vi "Calc ScaleFactor.vi"(8 "error in (no error)":errorcluster, 11 "[A/D Input]":dbl[][](array[numeric])) -> (0 "error out":errorcluster, 1 "ScaleFactorB":i32, 2 "ScaleFactorA":i32, 3 "Pass?":bool, 4 "May Pass Retest?":bool, 5 "GAINC":string, 6 "AssyScore":i32, 7 "PCBScore":i32, 9 "Pass/Fail #":dbl)   [LabVIEW 2013]
uses:
  <vilib>/Utility/NIReport.llb/NI_report.lvclass
  <vilib>/addons/_office/NI_ReportGenerationToolkit.lvlib
  InputScript states.ctl
  <vilib>/addons/_office/excel.llb/Excel Get Data ([dbl]).vi
  <vilib>/Utility/NIReport.llb/Excel/NI_Excel.lvclass
  <vilib>/addons/_office/excel.llb/Excel Easy Table (num).vi
  <vilib>/addons/_office/excel.llb/Excel Get Data (str).vi
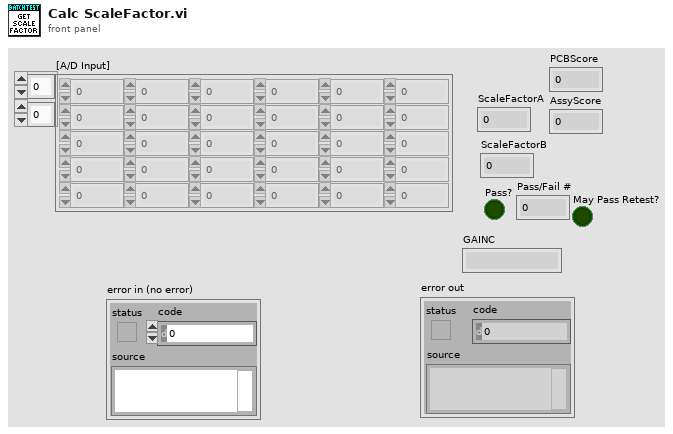
[diagram p1: front panel]
types:
  T1 = typedef "InputScript states.ctl" = enum16{"Open Template", "Setup parameters", "Read Input Script", "Close Template"}
  T2 = enum16{"maximized", "minimized", "normal", "no change"}
  T3 = enum16{"Standard Report", "HTML", "Word", "Excel"}
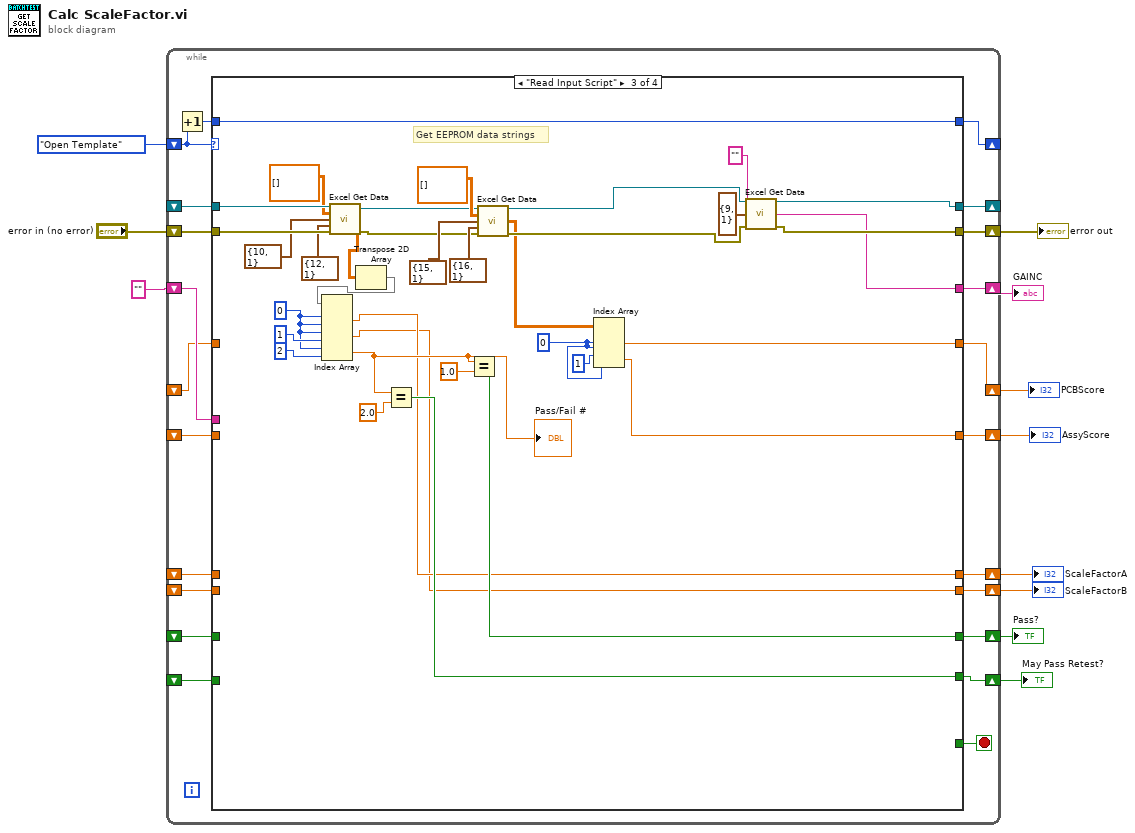
[diagram p0: block diagram]
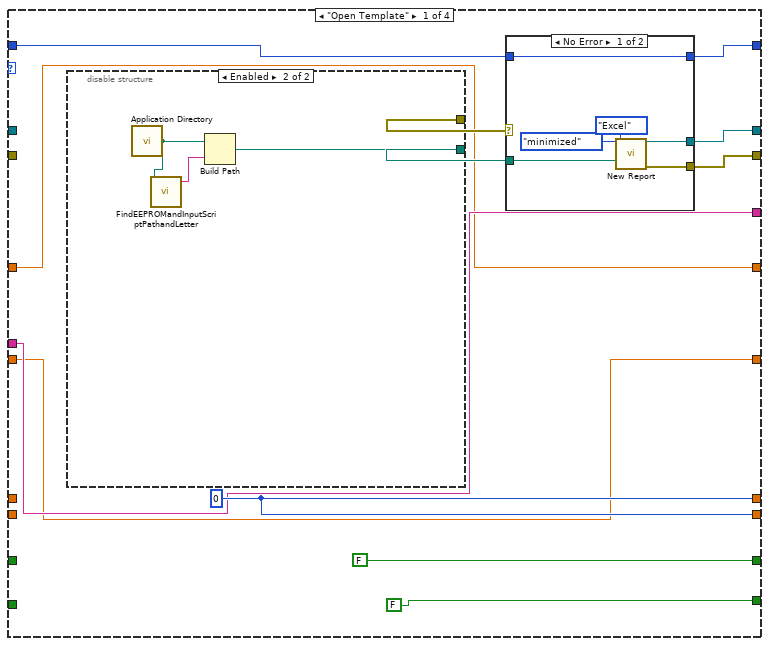
[diagram p2: hidden frame]
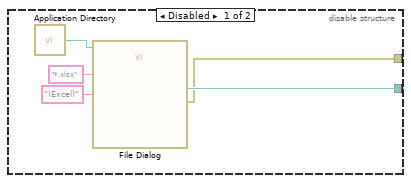
[diagram p3: hidden frame]
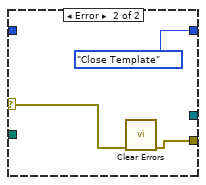
[diagram p4: hidden frame]
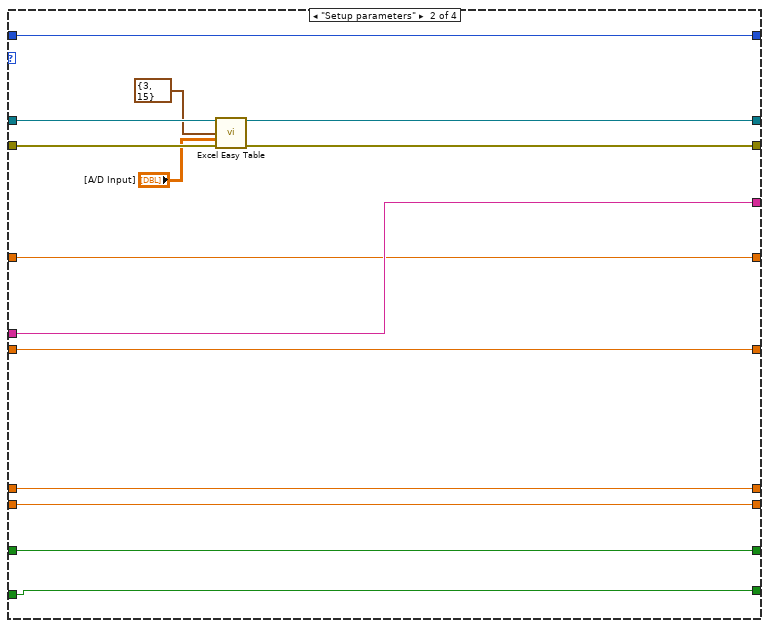
[diagram p5: hidden frame]
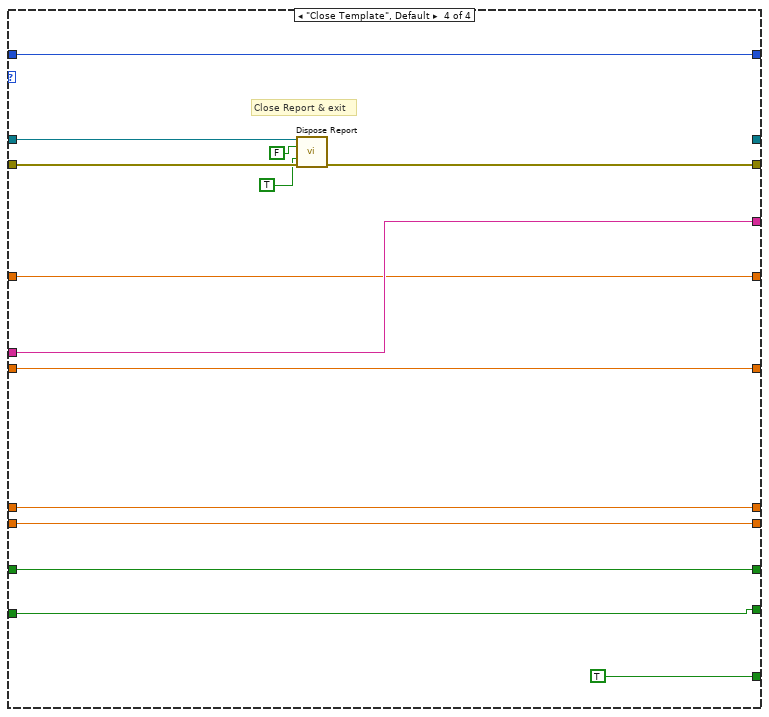
[diagram p6: hidden frame]
diagram:
  n1 = while {
    shift-right: [w32] -> _
    shift-left: _ -> [w31]
    shift-right: [w30] -> w9
    shift-left: "error in (no error)" -> [w29]
    shift-right: [w26] -> _
    shift-left: InputScript_states."Open Template" -> [w28]
    shift-right: [w25] -> w8
    shift-left: _ -> [w24]
    shift-right: [w23] -> w7
    shift-left: _ -> [w22]
    shift-right: [w21] -> w6
    shift-left: _ -> [w20]
    shift-right: [w19] -> w5
    shift-left: _ -> [w18]
    shift-right: [w17] -> w4
    shift-left: "" ("data") -> [w16]
    shift-right: [w15] -> w2
    shift-left: _ -> [w13]
    shift-right: [w14] -> w1
    shift-left: _ -> [w12]
    stop <- w33 stop-if-true
    n2 = Increment(x=w28) -> (x+1=w27:T1)
    n3 = case shown="\"Read Input Script\"" w28 {
      tunnel: [_ _ _ TRUE] -> w33
      tunnel: [w45 w68 w98 _] -> w32
      tunnel: w31 -> [_ w74 w111 w124]
      tunnel: [w44 w67 w99 w122] -> w30
      tunnel: w29 -> [_ w73 w110 w123]
      tunnel: w27 -> [w41 w76 w109 w120]
      tunnel: [w40 w76 w109 w120] -> w26
      tunnel: [w38 w75 w78 w119] -> w25
      tunnel: w24 -> [_ w75 _ w119]
      tunnel: [FALSE w70 w79 w118] -> w23
      tunnel: w22 -> [_ w70 _ w118]
      tunnel: [w38 w69 w77 w117] -> w21
      tunnel: w20 -> [_ w69 _ w117]
      tunnel: [FALSE w66 w101 w115] -> w19
      tunnel: w18 -> [_ w66 _ w115]
      tunnel: [w36 w65 w96 w114] -> w17
      tunnel: w16 -> [w36 w65 _ w114]
      tunnel: [w35 w64 w87 w113] -> w15
      tunnel: [w34 w63 w86 w112] -> w14
      tunnel: w13 -> [w35 w64 _ w113]
      tunnel: w12 -> [w34 w63 _ w112]
      frame "Open Template" {
        w38 = u8 0 ("ScaleFactor")
        n4 = disable-structure shown="Enabled" {
          disable-tunnel: [w47 w53] -> w43
          disable-tunnel: [w46 _] -> w42
          frame Disabled {
            n5 = call <vilib>:"Application Directory.vi"() -> ("Application Directory"=w48:path)
            n6 = call "File Dialog"("start path"=w48, "pattern (all files)"="*.xlsx", "pattern label"="(Excel)") -> ("selected path"=w47:path, "error out"=w46:errorcluster)  [unwired: 9 in, 2 out]
          }
          frame Enabled {
            n7 = call <vilib>:"Application Directory.vi"() -> ("Application Directory"=w52:path)
            n8 = call "FindEEPROMandInputScriptPathandLetter.vi"("path"=w52) -> ("EEPROM File"=w51:string)  [unwired: 3 in, 3 out]
            n9 = Build Path(base path=w52, name or relative path=w51) -> (appended path=w53:path)
          }
        }
        n10 = case shown="No Error" w42 {
          selector: w42 -> [_ w62]
          tunnel: [w58 _] -> w45
          tunnel: [w57 w61] -> w44
          tunnel: w43 -> [w56 _]
          tunnel: w41 -> [w55 _]
          tunnel: [w55 InputScript_states."Close Template"] -> w40
          frame No Error {
            n11 = call <vilib>:"New Report.vi"("window state (normal)"=T2."minimized", "report type"=T3."Excel", "template (empty)"=w56) -> ("report out"=w58:refnum<class "NI_report.lvclass">, "error out"=w57:errorcluster)  [unwired: 11 in]
          }
          frame Error {
            n12 = call <vilib>:"Clear Errors.vi"("error in (no error)"=w62) -> ("error out"=w61:errorcluster)  [unwired: 5 in, 1 out]
          }
        }
      }
      frame "Setup parameters" {
        n13 = call-poly <vilib>:"Excel Easy Table.vi"("report in"=w74, "start (0, 0)"=cluster{"row":i32, "column":i32} {"row"=3, "column"=15} ("start (-1, -1)"), "text data"="[A/D Input]", "error in (no error)"=w73) -> ("report out"=w68:refnum<class "NI_report.lvclass">, "error out"=w67:errorcluster)  [unwired: 7 in, 3 out]
      }
      frame "Read Input Script" {
        w84 = 0 ("index (row)")
        w104 = 0 ("index (row)")
        # "Get EEPROM data strings"
        n14 = call-poly <vilib>:"Excel Get Data.vi"("report in"=w111, "data type"=dbl[][] [], "start (-1, -1)"=cluster{"row":i32, "column":i32} {"row"=10, "column"=1}, "end (-1, -1)"=cluster{"row":i32, "column":i32} {"row"=12, "column"=1}, "error in (no error)"=w110) -> ("report out"=w92:refnum<class "NI_report.lvclass">, "data"=w83:dbl[][], "error out"=w91:errorcluster)  [unwired: 8 in]
        n15 = Transpose 2D Array(2D array=w83) -> (transposed array=w82:dbl[][])
        n16 = Index Array(array=w82, index (row) #1=w104, index (col) #1=w104, index (row) #2=w104, index (col) #2=1 ("disabled index (col)"), index (row) #3=w104, index (col) #3=2 ("disabled index (col)")) -> (element #1=w78:dbl, element #2=w77:dbl, element #3=w81:dbl)
        "Pass/Fail #" <- w81
        n17 = Equal?(x=w81, y=2.0) -> (x = y?=w101:bool)
        n18 = Equal?(x=w81, y=1.0) -> (x = y?=w79:bool)
        n19 = call-poly <vilib>:"Excel Get Data.vi"("report in"=w92, "data type"=dbl[][] [], "start (-1, -1)"=cluster{"row":i32, "column":i32} {"row"=15, "column"=1}, "end (-1, -1)"=cluster{"row":i32, "column":i32} {"row"=16, "column"=1}, "error in (no error)"=w91) -> ("report out"=w90:refnum<class "NI_report.lvclass">, "data"=w88:dbl[][], "error out"=w89:errorcluster)  [unwired: 8 in]
        n20 = Index Array(array=w88, index (row) #1=w84, index (col) #1=w84, index (row) #2=1 ("disabled index (col)"), index (col) #2=w84) -> (element #1=w87:dbl, element #2=w86:dbl)
        n21 = call-poly <vilib>:"Excel Get Data.vi"("report in"=w90, "data type"="", "start (0, 0)"=cluster{"start row":i32, "start column":i32} {"start row"=9, "start column"=1}, "error in (no error)"=w89) -> ("report out"=w98:refnum<class "NI_report.lvclass">, "data"=w96:string, "error out"=w99:errorcluster)  [unwired: 9 in]
      }
      frame "Close Template", Default {
        # "Close Report & exit"
        n22 = call-dynamic "Dispose Report.vi"("report in"=w124, "wait until printing completed? (T)"=FALSE, "save changes? (F)"=TRUE, "error in (no error)"=w123) -> ("error out"=w122:errorcluster)  [unwired: 11 in]
      }
    }
  }
  "error out" <- w9
  "ScaleFactorA" <- w8
  "Pass?" <- w7
  "ScaleFactorB" <- w6
  "May Pass Retest?" <- w5
  "GAINC" <- w4
  "PCBScore" <- w2
  "AssyScore" <- w1
